vi "test Cant Retry A Timeout If Cancel On Timeout Is Set.vi"(8 "error in (no error)":errorcluster, 11 "TestCase in":refnum<class "Futures Tests.lvclass">) -> (0 "error out":errorcluster, 3 "TestCase out":refnum<class "Futures Tests.lvclass">)   [LabVIEW 2017, in "Futures Tests.lvclass"]
uses:
  Futures Tests.lvclass
  <vilib>/addons/_JKI Toolkits/VI Tester/TestCase.llb/TestCase.lvclass
  Futures/Futures.lvlib
  Futures/Future/Future.lvclass
  Futures/Promise/Promise.lvclass
  C:/Program Files (x86)/National Instruments/LabVIEW 2017/vi.lib/addons/_JKI Toolkits/VI Tester/TestCase.llb/TestCase.lvclass
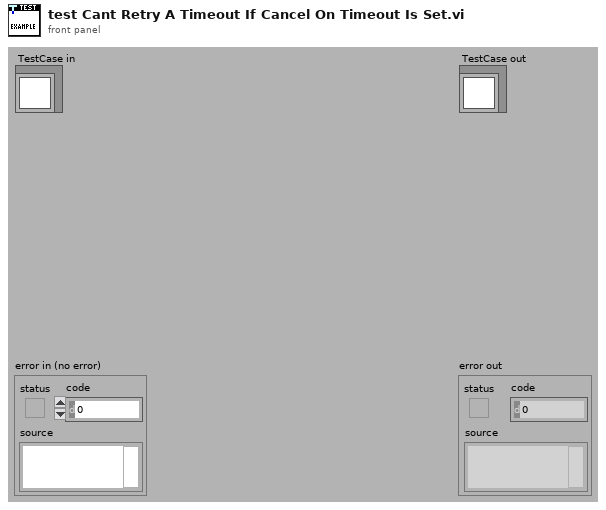
[diagram p1: front panel]
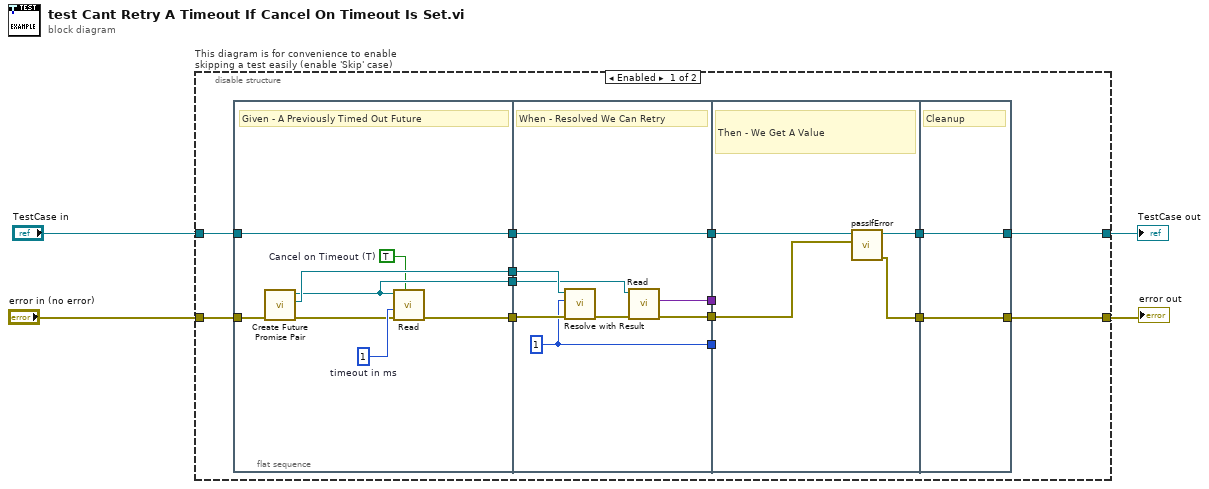
[diagram p0: block diagram]
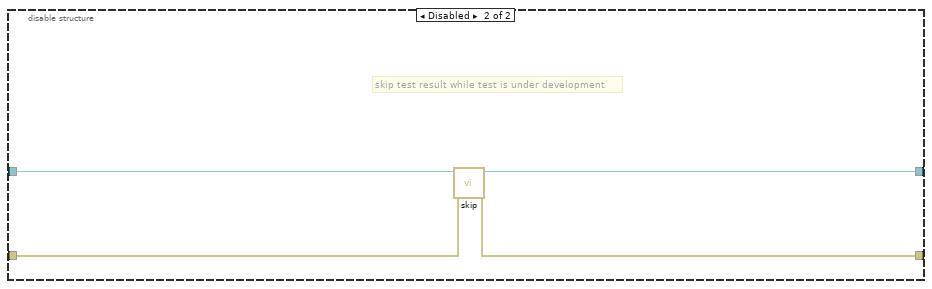
[diagram p2: hidden frame]
diagram:
  n1 = disable-structure "This diagram is for convenience to enable skipping a test easily (enable 'Skip' case)" shown="Enabled" {
    disable-tunnel: "TestCase in" -> [w14 w44]
    disable-tunnel: [w12 w42] -> w1
    disable-tunnel: [w11 w43] -> w3
    disable-tunnel: "error in (no error)" -> [w13 w41]
    frame Enabled {
      n2 = flat-sequence {
        tunnel: w13 -> [w25]
        tunnel: w14 -> [w26]
        tunnel: [w26] -> w18
        tunnel: [w22] -> w10
        tunnel: [w21] -> w9
        tunnel: [w20] -> w8
        tunnel: [w34] -> w17
        tunnel: w18 -> [w34]
        tunnel: w10 -> [w33]
        tunnel: w9 -> [w31]
        tunnel: w8 -> [w30]
        tunnel: [w29] -> w7
        tunnel: [w28] -> w6
        tunnel: [w27] -> w5
        tunnel: [w37] -> w16
        tunnel: [w36] -> w15
        tunnel: w17 -> [w38]
        tunnel: w7 -> [w35]
        tunnel: w6 -> [_]
        tunnel: w5 -> [_]
        tunnel: [w39] -> w11
        tunnel: [w40] -> w12
        tunnel: w16 -> [w40]
        tunnel: w15 -> [w39]
        frame #0 {
          w19 = TRUE  # Cancel on Timeout (T)
          w24 = 1  # timeout in ms
          # "Given - A Previously Timed Out Future"
          n3 = call "Create Future Promise Pair.vi"("error in (no error)"=w25) -> ("error out"=w23:errorcluster, "Promise out"=w21:refnum<class "Promise.lvclass">, "Future out"=w20:refnum<class "Future.lvclass">)  [unwired: 8 in]
          n4 = call "Read.vi"("Cancel on Timeout (T)"=w19, "error in (no error)"=w23, "timeout in ms (60 sec)"=w24, "Future in"=w20) -> ("error out"=w22:errorcluster)  [unwired: 4 in, 3 out]
        }
        frame #1 {
          w27 = 1
          # "When - Resolved We Can Retry"
          n5 = call "Resolve with Result.vi"("error in (no error)"=w33, "Result"=w27, "Promise in"=w31) -> ("error out"=w32:errorcluster)  [unwired: 8 in]
          n6 = call "Read.vi"("error in (no error)"=w32, "Future in"=w30) -> ("error out"=w29:errorcluster, "Result value"=w28:variant)  [unwired: 6 in, 2 out]
        }
        frame #2 {
          # "Then - We Get A Value"
          n7 = call-dynamic "passIfError.vi"("error"=w35, "TestCase in"=w38) -> ("error out"=w36:errorcluster, "TestCase out"=w37:refnum<class "Futures Tests.lvclass">)  [unwired: 8 in]
        }
        frame #3 {
          # "Cleanup"
        }
      }
    }
    frame Disabled {
      # "skip test result while test is under development"
      n8 = call <vilib>:"skip.vi"("error in (no error)"=w41, "TestCase in"=w44) -> ("error out"=w43:errorcluster, "TestCase out"=w42:refnum<class "Futures Tests.lvclass">)  [unwired: 8 in]
    }
  }
  "error out" <- w3
  "TestCase out" <- w1
